vi "Updater Convert TDMS File 4.3 to 5.0.vi"(8 "error in (no error)":errorcluster, 10 "Map IndexName to FieldId":T1(array[cluster]), 11 "TDMS Path":path) -> (0 "error out":errorcluster, 3 "Conversion Time (ms)":u32)   [LabVIEW 2011]
uses:
  Summitek EXT/OpenG EXT/file/file.llb/Strip Path Extension - String__ogtk.vi
  Summitek EXT/OpenG EXT/file/file.llb/Convert File Extension (Path)__ogtk.vi
panel:
  out "Group Names":string[](array[string])
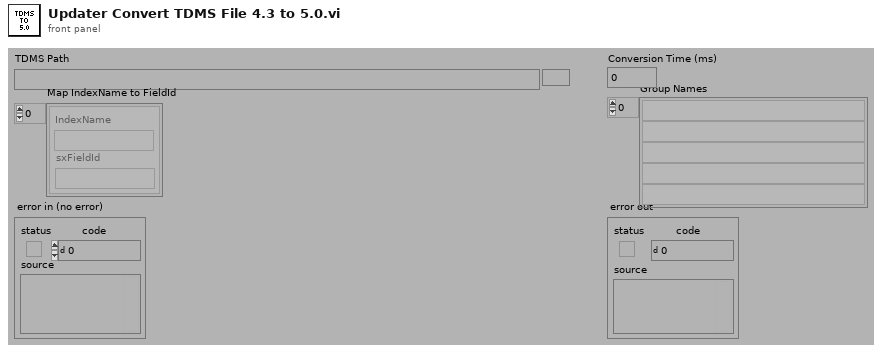
[diagram p1: front panel]
types:
  T1 = cluster{"IndexName":string, "sxFieldId":string}[]
  T2 = enum16{"open", "open or create", "create or replace", "create", "open (read-only)"}
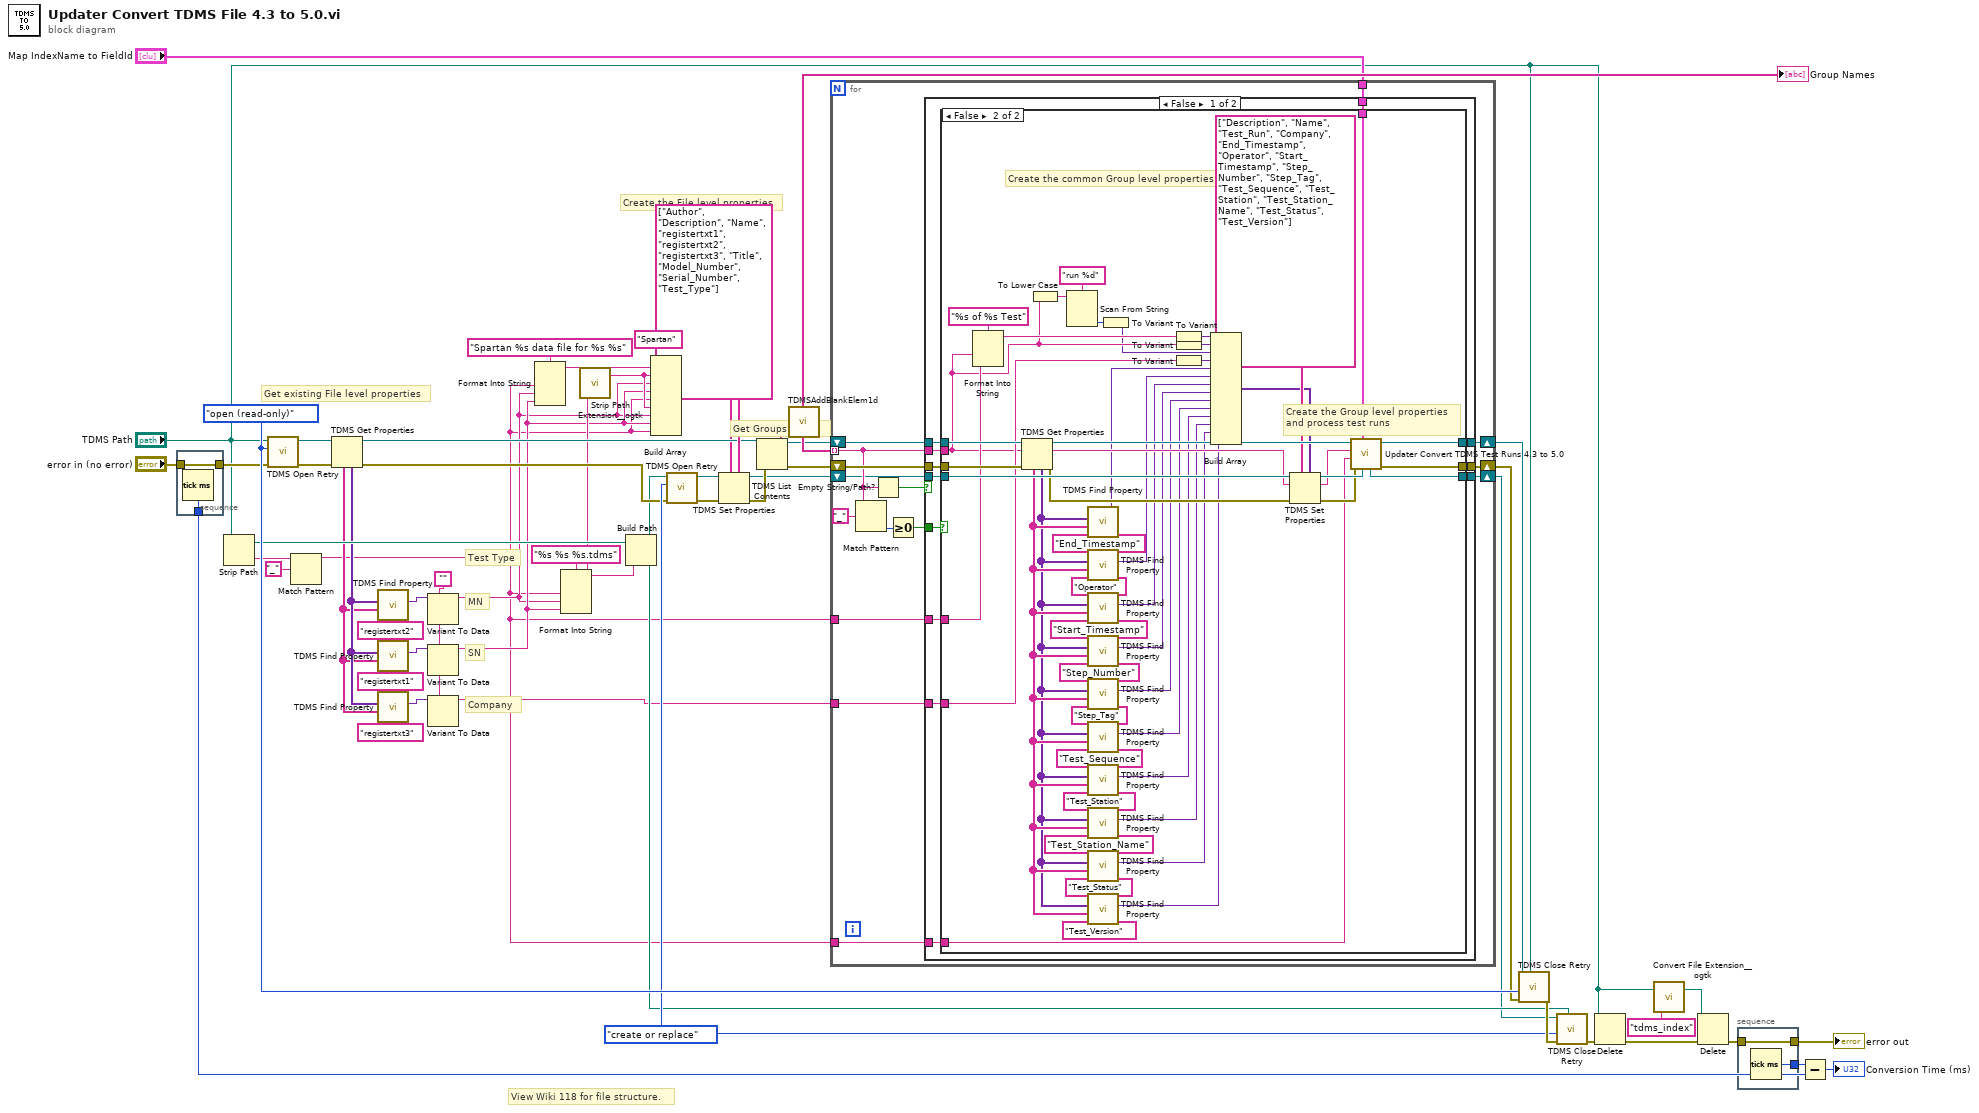
[diagram p0: block diagram]
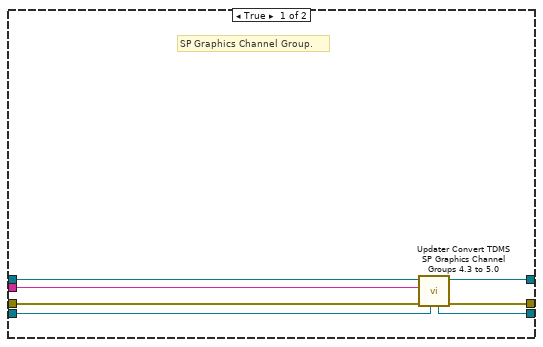
[diagram p2: hidden frame]
diagram:
  w9 = ""
  w46 = T2."create or replace" ("operation (0:open)")
  w56 = T2."open (read-only)" ("operation (0:open)")
  # "Company"
  # "Get Groups (Runs)"
  # "Get existing File level properties"
  # "View Wiki 118 for file structure."
  # "MN"
  # "SN"
  # "Test Type"
  # "Create the File level properties"
  n1 = stacked-sequence {
    tunnel: "error in (no error)" -> [w58]
    tunnel: [w58] -> w35
    tunnel: [w57] -> w32
    frame #0 {
      n2 = Tick Count (ms)() -> (millisecond timer value=w57:u32)
    }
  }
  n3 = Strip Path(path="TDMS Path") -> (stripped path=w50:path, name=w43:string)
  n4 = call "TDMS Open Retry.vi"("error in (no error)"=w35, "Operation (0:open)"=w56, "Path"="TDMS Path") -> ("error out"=w44:errorcluster, "TDMS File Ref"=w55:refnum<k34>)  [unwired: 1 in, 6 out]
  n5 = Match Pattern(string=w43, regular expression="_") -> (before substring=w3:string)  [unwired: 4 out]
  n6 = TDMS Get Properties(8:w44, 11:w55) -> (0:w39:errorcluster, 3:w48:refnum<k34>, 4:w17:variant[], 6:w16:string[])  [unwired: 1 in, 5 out]
  n7 = call "TDMS Find Property.vi"("Property Name"="registertxt2" ("element"), "Property Names"=w16, "Property Values"=w17) -> ("Property Value"=w10:variant)  [unwired: 5 out]
  n8 = call "TDMS Find Property.vi"("Property Name"="registertxt1" ("element"), "Property Names"=w16, "Property Values"=w17) -> ("Property Value"=w13:variant)  [unwired: 5 out]
  n9 = call "TDMS Find Property.vi"("Property Name"="registertxt3" ("element"), "Property Names"=w16, "Property Values"=w17) -> ("Property Value"=w15:variant)  [unwired: 5 out]
  n10 = Variant To Data(type=w9, Variant=w10) -> (data=w11:string)  [unwired: 1 in, 1 out]
  n11 = Variant To Data(type=w9, Variant=w13) -> (data=w12:string)  [unwired: 1 in, 1 out]
  n12 = Variant To Data(type=w9, Variant=w15) -> (data=w14:string)  [unwired: 1 in, 1 out]
  n13 = Format Into String(format string="Spartan %s data file for %s %s", w3, w11, w12) -> (resulting string=w27:string)  [unwired: 2 in, 1 out]
  n14 = Format Into String(format string="%s %s %s.tdms", w3, w11, w12) -> (resulting string=w26:string)  [unwired: 2 in, 1 out]
  n15 = call-poly "Strip Path Extension__ogtk.vi"("path"=w26) -> ("root"=w25:string)  [unwired: 1 out]
  n16 = Build Path(base path=w50, name or relative path=w26) -> (appended path=w30:path)
  n17 = Build Array("Spartan" ("element"), w27, w25, w11, w12, w3, w25, w11, w12, w3) -> (w49:string[])
  n18 = call "TDMS Open Retry.vi"("error in (no error)"=w39, "Operation (0:open)"=w46, "Path"=w30) -> ("error out"=w38:errorcluster, "TDMS File Ref"=w37:refnum<k34>)  [unwired: 1 in, 6 out]
  n19 = TDMS Set Properties(5:w49, 7:string[] ["Author", "Description", "Name", "registertxt1", "registertxt2", "registertxt3", "Title", "Model_Number", "Serial_Number", "Test_Type"], 8:w38, 11:w37) -> (0:w54:errorcluster, 3:w24:refnum<k34>)  [unwired: 4 out]
  n20 = TDMS List Contents(4:w54, 7:w48) -> (0:w53:errorcluster, 2:w2:string[], 3:w22:refnum<k34>)  [unwired: 2 out]
  n21 = call <vilib>:"TDMSAddBlankElem1d.vi"("input string array"=w2) -> ("output string array with blank element at the beginning"=w52:string[])
  "Group Names" <- w52
  n22 = for {
    shift-right: [w71] -> w51
    shift-left: w53 -> [w72]
    tunnel: w52 -> [w69] mode=indexing
    tunnel: w3 -> [w67]
    tunnel: "Map IndexName to FieldId" -> [w66]
    tunnel: w14 -> [w64]
    shift-right: [w61] -> w21
    shift-left: w22 -> [w73]
    shift-right: [w60] -> w23
    shift-left: w24 -> [w65]
    tunnel: w3 -> [w59]
    n23 = Match Pattern(string=w69, regular expression="_") -> (offset past match=w68:i32)  [unwired: 4 out]
    n24 = Empty String/Path?(string/path=w69) -> (empty?=w62:bool)
    n25 = Greater Or Equal To 0?(x=w68) -> (x >= 0?=w63:bool)
    n26 = case shown="False" w62 {
      tunnel: w73 -> [w85 w143]
      tunnel: w72 -> [w84 w144]
      tunnel: [w83 w144] -> w71
      tunnel: w69 -> [w82 _]
      tunnel: w67 -> [w81 _]
      tunnel: w66 -> [w80 _]
      tunnel: w65 -> [w79 w142]
      tunnel: w64 -> [w78 _]
      tunnel: w63 -> [w77 _]
      tunnel: [w76 w143] -> w61
      tunnel: [w75 w142] -> w60
      tunnel: w59 -> [w74 _]
      frame False {
        n27 = case shown="False" w77 {
          tunnel: w85 -> [w90 w140]
          tunnel: w84 -> [w92 w137]
          tunnel: w82 -> [w89 w97]
          tunnel: [w88 w133] -> w83
          tunnel: w81 -> [_ w101]
          tunnel: w80 -> [_ w141]
          tunnel: w79 -> [w91 w139]
          tunnel: w78 -> [_ w108]
          tunnel: [w87 w109] -> w76
          tunnel: [w86 w110] -> w75
          tunnel: w74 -> [_ w102]
          frame True {
            # "SP Graphics Channel Group."
            n28 = call "Updater Convert TDMS SP Graphics Channel Groups 4.3 to 5.0.vi"("New TDMS File In"=w91, "error in (no error)"=w92, "Group Name In"=w89, "Source TDMS File In"=w90) -> ("error out"=w88:errorcluster, "Source TDMS File Out"=w87:refnum<k34>, "New TDMS File Out"=w86:refnum<k34>)  [unwired: 5 out]
          }
          frame False {
            # "Create the common Group level properties"
            # "Create the Group level properties\nand process test runs"
            n29 = Format Into String(format string="%s of %s Test", w97, w102) -> (resulting string=w107:string)  [unwired: 2 in, 1 out]
            n30 = TDMS Get Properties(8:w137, 10:w97, 11:w140) -> (0:w135:errorcluster, 2:w132:string, 4:w118:variant[], 6:w119:string[])  [unwired: 1 in, 4 out]
            n31 = To Lower Case(string=w97) -> (all lower case string=w93:string)
            n32 = Scan From String(format string="run %d", input string=w93) -> (output 1=w95:i32)  [unwired: 2 in, 4 out]
            n33 = call "TDMS Find Property.vi"("Property Name"="End_Timestamp" ("element"), "Property Names"=w119, "Property Values"=w118) -> ("Property Value"=w128:variant)  [unwired: 5 out]
            n34 = call "TDMS Find Property.vi"("Property Name"="Operator" ("element"), "Property Names"=w119, "Property Values"=w118) -> ("Property Value"=w117:variant)  [unwired: 5 out]
            n35 = call "TDMS Find Property.vi"("Property Name"="Start_Timestamp" ("element"), "Property Names"=w119, "Property Values"=w118) -> ("Property Value"=w116:variant)  [unwired: 5 out]
            n36 = call "TDMS Find Property.vi"("Property Name"="Step_Number" ("element"), "Property Names"=w119, "Property Values"=w118) -> ("Property Value"=w115:variant)  [unwired: 5 out]
            n37 = call "TDMS Find Property.vi"("Property Name"="Step_Tag" ("element"), "Property Names"=w119, "Property Values"=w118) -> ("Property Value"=w114:variant)  [unwired: 5 out]
            n38 = call "TDMS Find Property.vi"("Property Name"="Test_Sequence" ("element"), "Property Names"=w119, "Property Values"=w118) -> ("Property Value"=w113:variant)  [unwired: 5 out]
            n39 = call "TDMS Find Property.vi"("Property Name"="Test_Station" ("element"), "Property Names"=w119, "Property Values"=w118) -> ("Property Value"=w112:variant)  [unwired: 5 out]
            n40 = call "TDMS Find Property.vi"("Property Name"="Test_Station_Name" ("element"), "Property Names"=w119, "Property Values"=w118) -> ("Property Value"=w105:variant)  [unwired: 5 out]
            n41 = call "TDMS Find Property.vi"("Property Name"="Test_Status" ("element"), "Property Names"=w119, "Property Values"=w118) -> ("Property Value"=w111:variant)  [unwired: 5 out]
            n42 = call "TDMS Find Property.vi"("Property Name"="Test_Version" ("element"), "Property Names"=w119, "Property Values"=w118) -> ("Property Value"=w103:variant)  [unwired: 5 out]
            n43 = To Variant(anything=w95) -> (Variant=w94:variant)
            n44 = To Variant(anything=w107) -> (Variant=w100:variant)
            n45 = To Variant(anything=w97) -> (Variant=w98:variant)
            n46 = To Variant(anything=w108) -> (Variant=w99:variant)
            n47 = Build Array(w100, w98, w94, w99, w128, w117, w116, w115, w114, w113, w112, w105, w111, w103) -> (w134:variant[])
            n48 = TDMS Set Properties(5:w134, 7:string[] ["Description", "Name", "Test_Run", "Company", "End_Timestamp", "Operator", "Start_Timestamp", "Step_Number", "Step_Tag", "Test_Sequence", "Test_Station", "Test_Station_Name", "Test_Status", "Test_Version"], 8:w135, 10:w132, 11:w139) -> (0:w129:errorcluster, 2:w130:string, 3:w131:refnum<k34>)  [unwired: 2 out]
            n49 = call "Updater Convert TDMS Test Runs 4.3 to 5.0.vi"("New TDMS File In"=w131, "Map IndexName to FieldId"=w141, "error in (no error)"=w129, "Test Type"=w101, "Group Name In"=w130, "Source TDMS File In"=w140) -> ("error out"=w133:errorcluster, "Source TDMS File Out"=w109:refnum<k34>, "New TDMS File Out"=w110:refnum<k34>)  [unwired: 3 out]
          }
        }
      }
      frame True {
        # "Blank is group that holds file data"
      }
    }
  }
  n50 = call "TDMS Close Retry.vi"("TDMS Path"="TDMS Path", "error in (no error)"=w51, "Operation (0:open)"=w56, "TDMS File Ref"=w21) -> ("error out"=w47:errorcluster)  [unwired: 1 in, 6 out]
  n51 = call "TDMS Close Retry.vi"("TDMS Path"=w30, "error in (no error)"=w47, "Operation (0:open)"=w46, "TDMS File Ref"=w23) -> ("error out"=w1:errorcluster)  [unwired: 1 in, 6 out]
  n52 = Delete(path (use dialog)="TDMS Path", error in=w1) -> (error out=w8:errorcluster)  [unwired: 5 out]
  n53 = call-poly "Convert File Extension__ogtk.vi"("new ending (none)"="tdms_index", "file name"="TDMS Path") -> ("new filename"=w5:path)  [unwired: 1 out]
  n54 = Delete(path (use dialog)=w5, error in=w8) -> (error out=w7:errorcluster)  [unwired: 5 out]
  n55 = stacked-sequence {
    tunnel: w7 -> [w146]
    tunnel: [w146] -> w34
    tunnel: [w145] -> w33
    frame #0 {
      n56 = Tick Count (ms)() -> (millisecond timer value=w145:u32)
    }
  }
  "error out" <- w34
  n57 = Subtract(x=w33, y=w32) -> (x-y=→"Conversion Time (ms)":u32)
